vi "Load Plugin Prepare.vi"(6 "Version String":string, 8 "error in (no error)":errorcluster, 9 "Unique Name":string, 10 "Plugin Type":string="CIFTemplatePlugin", 11 "CIFPluginManager in":refnum<class "CIFPluginManager.lvclass">) -> (0 "error out":errorcluster, 1 "Unique Name (dup)":string, 2 "Matching Plugin":T1, 5 "path":string)   [LabVIEW 2021, in "CIFPluginManager.lvclass"]
doc: "This prepares the loading action. Because the VI server process can be slow it is moved outside of the Load Plugin Prepare process to the Load Plugin Action. The prepare will detect most common configuration errors. This allows the UI to get any configuration errors returned but not need to wait for the full load to complete."
uses:
  CIFPluginManager.lvclass
  typedef/Discovered Plugin.ctl
  <vilib>/CIF Foundation/CIF Core/CIFCore/Common/Typedef/Version.ctl
  typedef/Plugin Metadata.ctl
  typedef/Loader Type.ctl
  <vilib>/CIF Foundation/CIF Core/CIFCore/Common/Typedef/Errors.ctl
  CIFPluginManager.lvclass/CIFPluginManager.ctl
  <vilib>/CIF Foundation/CIF Utilities/Errors/Append Error Location.vi
  <vilib>/CIF Foundation/CIF Core/CIFCore/Common/CIFCoreCommon.lvlib
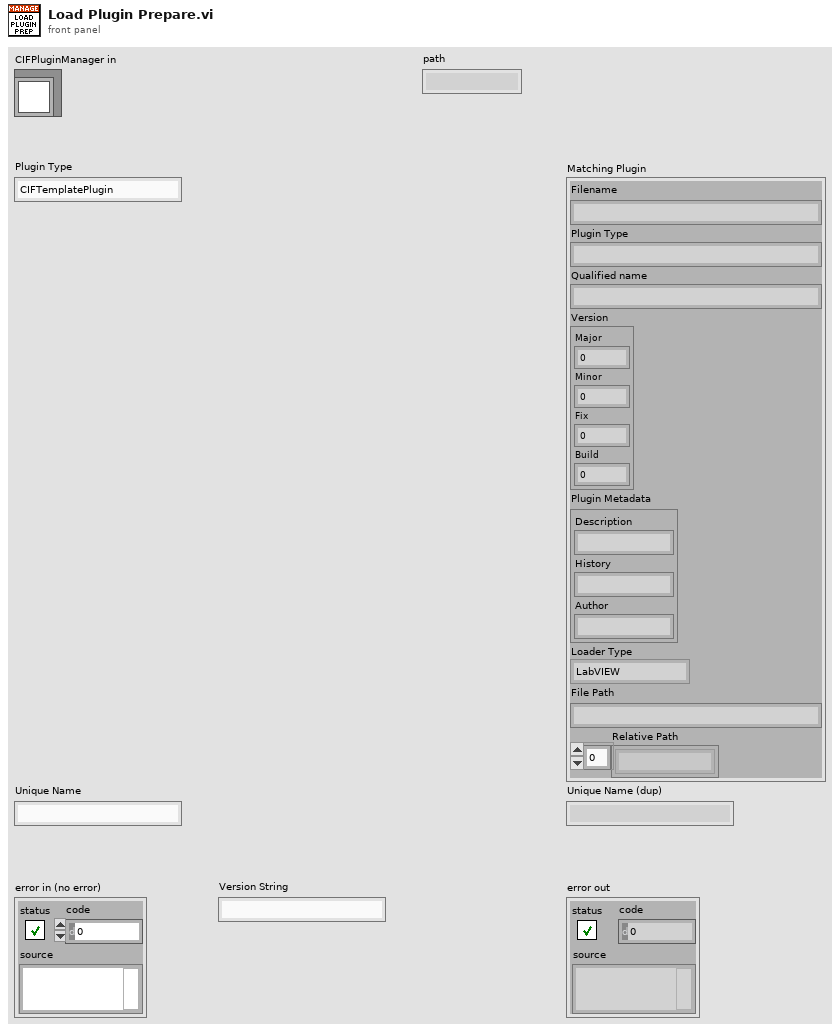
[diagram p1: front panel]
types:
  T1 = typedef "CIFPluginManager.lvclass/Discovered Plugin.ctl" = cluster{"Filename":string, "Plugin Type":string, "Qualified name":string, "Version":T2, "Plugin Metadata":T3, "Loader Type":T4, "File Path":string, "Relative Path":string[]}
  T2 = typedef "CIFCoreCommon.lvlib/Version.ctl" = cluster{"Major":i32, "Minor":i32, "Fix":i32, "Build":i32}
  T3 = typedef "CIFPluginManager.lvclass/Plugin Metadata.ctl" = cluster{"Description":string, "History":string, "Author":string}
  T4 = typedef "CIFPluginManager.lvclass/Loader Type.ctl" = enum16{"LabVIEW"}
  T5 = typedef "CIFCoreCommon.lvlib/Errors.ctl" = enum16{"Invalid Clock ID", "Long Sleep", "gRPC Server Not Found", "Config Parse", "Timestamp Wrap", "Delayed Execution", "Duplicate Channel", "Missing Channel", "Incorrect Type", "Flatten Error", "Unflatten Data", "Unique Name", "Plugin Not Found", "Plugin Type Not Found", "Plugin Version Not Found", "Manager Not Found", "Numerical Issue", "Time Jump", "Clock ID Match", "Channel Length", "Plugin Connection", "gRPC Server Connection", "PPL Name Match", "Build", "Config Log Parse", "Plugin Load", "UI Subpanel Load", "Python Name", "Invalid Name", "Unable to Change Ch Buffer", "Failed Kill", "Failed SysExec", "Function Not Implemented", "Load Timeout"}
  T6 = typedef "CIFPluginManager.lvclass/Plugin Management Data Map.ctl" = map{string, T7}
  T7 = typedef "CIFPluginManager.lvclass/Plugin Management Data.ctl" = cluster{"Unique Name":string, "Plugin Type":string, "gRPC Port":i32, "gRPC ID":T8, "Loader Type":T4, "Loader":string, "Version":T2, "Load Timestamp":i64, "Unload Timestamp":i64, "Unloading":bool, "Ready for removal":bool, "status":T9, "channels":T18}
  T8 = typedef "grpc-lvsupport-release.lvlib/grpcId.ctl" = u64
  T9 = typedef "CIF_Manager_server.lvlib/cif_management_common_PluginStatusData.ctl" = cluster{"state":T10, "timing_statistics":T11, "fifo_statistics":T13, "error":T14, "monitor_doubles":T15, "monitor_u64s":T16, "monitor_i64s":T17}
  T10 = typedef "CIF_Manager_server.lvlib/cif_management_common_PluginStatusData_PluginState.ctl" = enum32{"PLUGINSTATE_UNKNOWN", "PLUGINSTATE_CREATING", "PLUGINSTATE_LISTENING", "PLUGINSTATE_RUNNING", "PLUGINSTATE_CLEANINGUP", "PLUGINSTATE_DESTROYING"}
  T11 = typedef "CIF_Manager_server.lvlib/cif_management_common_TimingStatistics.ctl" = cluster{"period":T12, "wake_error":T12, "execute":T12, "housekeep":T12, "idle":T12, "cleanup":T12, "custom_1":T12, "custom_2":T12}
  T12 = typedef "CIF_Manager_server.lvlib/cif_common_TimingStats.ctl" = cluster{"max":i64, "min":i64, "avg":dbl}
  T13 = typedef "CIF_Manager_server.lvlib/cif_management_common_FifoStatistics.ctl" = cluster{"from_t0":T12, "from_previous_plugin":T12, "output_error":T12}
  T14 = typedef "CIF_Manager_server.lvlib/cif_management_common_Error.ctl" = cluster{"status":bool, "code":i32}
  T15 = typedef "CIF_Manager_server.lvlib/cif_management_common_MonitorDoubles.ctl" = cluster{"double_1":dbl, "double_2":dbl, "double_3":dbl, "double_4":dbl}
  T16 = typedef "CIF_Manager_server.lvlib/cif_management_common_MonitorU64.ctl" = cluster{"u64_1":u64, "u64_2":u64, "u64_3":u64, "u64_4":u64}
  T17 = typedef "CIF_Manager_server.lvlib/cif_management_common_MonitorI64.ctl" = cluster{"i64_1":i64, "i64_2":i64, "i64_3":i64, "i64_4":i64}
  T18 = typedef "CIF_Manager_server.lvlib/cif_management_common_Channels.ctl" = cluster{"channels":T19[]}
  T19 = typedef "CIF_Manager_server.lvlib/cif_management_common_Channel.ctl" = cluster{"name":string, "direction":T20, "type":string, "custom_config":u8[], "connected":bool, "connected_name":string, "forced":bool, "channel_pattern":T21}
  T20 = typedef "CIF_Manager_server.lvlib/cif_management_common_ChannelDirection.ctl" = enum32{"CHANNELDIRECTION_UNKNOWN", "CHANNELDIRECTION_PUBLISHER", "CHANNELDIRECTION_SUBSCRIBER"}
  T21 = typedef "CIF_Manager_server.lvlib/cif_management_common_ChannelPattern.ctl" = enum32{"CHANNELPATTERN_UNKNOWN", "CHANNELPATTERN_TAG", "CHANNELPATTERN_FIFO", "CHANNELPATTERN_MULTIFIFO", "CHANNELPATTERN_BACKPRESSUREFIFO"}
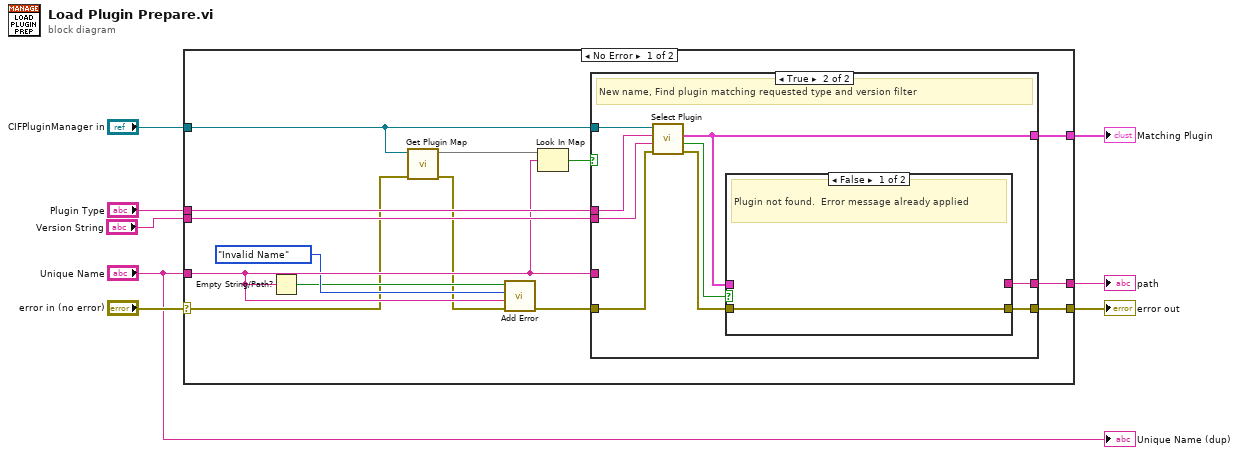
[diagram p0: block diagram]
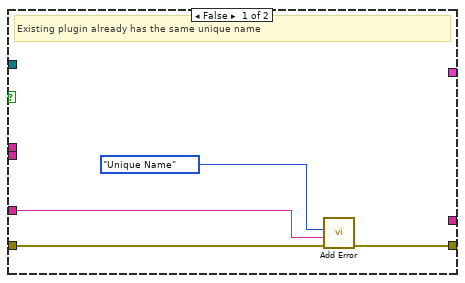
[diagram p2: hidden frame]
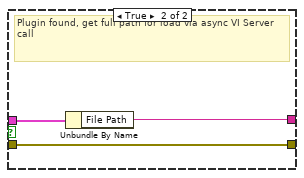
[diagram p3: hidden frame]
diagram:
  n1 = case shown="No Error" "error in (no error)" {
    selector: "error in (no error)" -> [w10 w40]
    tunnel: [w22 w40] -> w7
    tunnel: "CIFPluginManager in" -> [w11 _]
    tunnel: "Plugin Type" -> [w21 _]
    tunnel: "Unique Name" -> [w17 _]
    tunnel: "Version String" -> [w19 _]
    tunnel: [w14 _] -> w2
    tunnel: [w13 _] -> w1
    frame No Error {
      n2 = Empty String/Path?(string/path=w17) -> (empty?=w15:bool)
      n3 = call "Get Plugin Map.vi"("error in (no error)"=w10, "CIFPluginManager in"=w11) -> ("error out"=w9:errorcluster, "Plugin Map"=w12:T6)  [unwired: 8 in]
      n4 = call <vilib>:"Add Error.vi"("error in (no error)"=w9, "String to Append"=w17, "Error"=Errors."Invalid Name", "Insert Error"=w15) -> ("error out"=w18:errorcluster)  [unwired: 7 in]
      n5 = Look In Map(map=w12, key=w17) -> (key not found?=w20:bool)  [unwired: 1 in, 1 out]
      n6 = case shown="True" w20 {
        tunnel: w18 -> [w26 w31]
        tunnel: [w23 w35] -> w22
        tunnel: w21 -> [_ w33]
        tunnel: w17 -> [w24 _]
        tunnel: w11 -> [_ w34]
        tunnel: w19 -> [_ w32]
        tunnel: [_ w27] -> w14
        tunnel: [_ w28] -> w13
        frame False {
          # "Existing plugin already has the same unique name"
          n7 = call <vilib>:"Add Error.vi"("error in (no error)"=w26, "String to Append"=w24, "Error"=Errors."Unique Name") -> ("error out"=w23:errorcluster)  [unwired: 8 in]
        }
        frame True {
          # "New name, Find plugin matching requested type and version filter"
          n8 = call "Select Plugin.vi"("error in (no error)"=w31, "Version String"=w32, "Plugin Type"=w33, "CIFPluginManager in"=w34) -> ("error out"=w30:errorcluster, "Match found"=w29:bool, "Matching Plugin"=w27:T1)  [unwired: 5 in]
          n9 = case shown="False" w29 {
            tunnel: [w36 w37] -> w35
            tunnel: w30 -> [w36 w37]
            tunnel: w27 -> [_ w39]
            tunnel: [_ w38] -> w28
            frame False {
              # "Plugin not found.  Error message already applied"
            }
            frame True {
              # "Plugin found, get full path for load via async VI Server call"
              n10 = Unbundle By Name(w39) -> ("File Path"=w38:string)
            }
          }
        }
      }
    }
    frame Error {
    }
  }
  "error out" <- w7
  "Matching Plugin" <- w2
  "path" <- w1
  "Unique Name (dup)" <- "Unique Name"
